vi "SendActionNum.vi"(5 "Host port":u16, 6 "RT Actions":T1 {"Slow AO Array"."Duration, Gain, NewVal" format="%#_3g"}, 7 "Host IP":string, 8 "error in (no error)":errorcluster, 9 "action #":string, 10 "Host process":string, 11 "Queue in":T5) -> (0 "error out":errorcluster)   [LabVIEW 2018]
uses:
  <vilib>/NI/AMC/Message Queue.ctl
  <vilib>/NI/AMC/Message.ctl
  <vilib>/NI/Tools/Keyed Array/KeyedArray.ctl
  RT Actions.ctl
  ActionCluster.ctl
  Instructions_RT.ctl
  ParameterSubCluster.ctl
  <vilib>/NI/AMC/Create Single Message.vi
  <vilib>/NI/AMC/Update Message Routing Info.vi
  <vilib>/NI/AMC/Send Message.vi
  <vilib>/NI/AMC/AMC.lvlib
  <vilib>/NI/Tools/Keyed Array/Tools_KeyedArray.lvlib
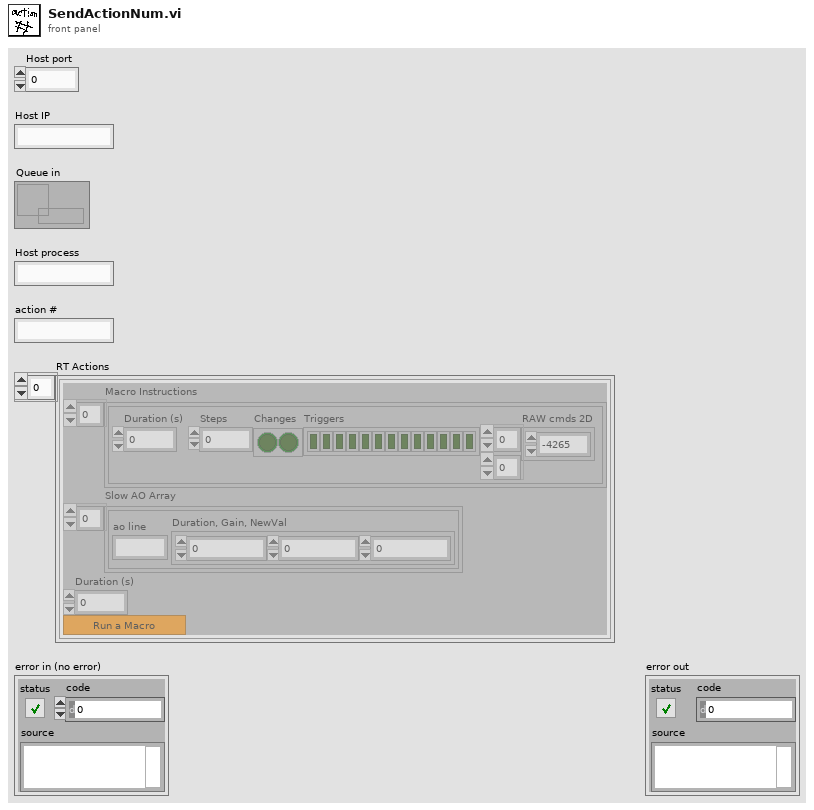
[diagram p1: front panel]
types:
  T1 = typedef "RT Actions.ctl" = T2[]
  T2 = typedef "ActionCluster.ctl" = cluster{"Macro Instructions":T3, "Slow AO Array":T4, "Duration (s)":dbl, "Toggle":bool}
  T3 = typedef "Instructions_RT.ctl" = cluster{"Duration (s)":dbl, "Steps":i32, "Changes":bool[], "Triggers":bool[], "RAW cmds 2D":i16[][]}[]
  T4 = typedef "ParameterSubCluster.ctl" = cluster{"ao line":string, "Duration, Gain, NewVal":dbl[]}[]
  T5 = typedef "AMC.lvlib/Message Queue.ctl" = refnum<queue>
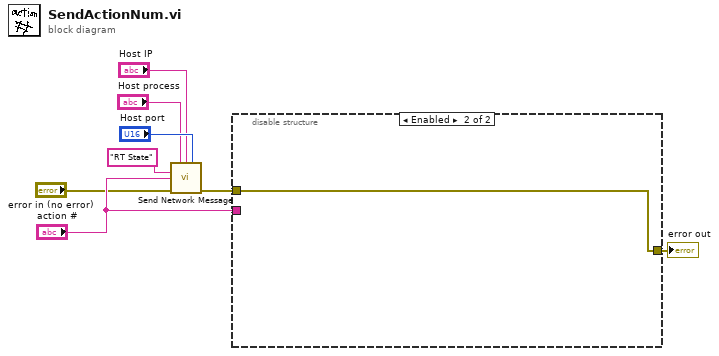
[diagram p0: block diagram]
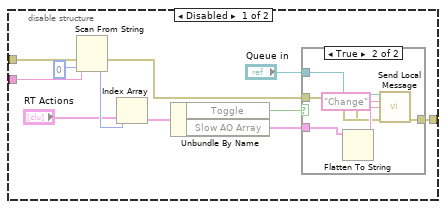
[diagram p2: hidden frame]
diagram:
  n1 = call <vilib>:"Send Network Message.vi"("receiver process"="Host process", "receiver host"="Host IP", "receiver port (0)"="Host port", "message name"="RT State", "message value"="action #", "error in"="error in (no error)") -> ("error out"=w2:errorcluster)  [unwired: 7 in, 2 out]
  n2 = disable-structure shown="Enabled" {
    disable-tunnel: "action #" -> [w19 _]
    disable-tunnel: w2 -> [w15 w27]
    disable-tunnel: [w9 w27] -> w1
    frame Disabled {
      n3 = Scan From String(input string=w19, error in=w15, default 1=u32 0 ("millisecond multiple")) -> (error out=w10:errorcluster, output 1=w18:u32)  [unwired: 2 in, 2 out]
      n4 = Index Array(array="RT Actions", index=w18) -> (element=w14:T2)
      n5 = Unbundle By Name(w14) -> ("Toggle"=w13:bool, "Slow AO Array"=w11:T4)
      n6 = case shown="True" w13 {
        tunnel: "Queue in" -> [_ w26]
        tunnel: w11 -> [_ w25]
        tunnel: w10 -> [w20 w22]
        tunnel: [w20 w21] -> _
        tunnel: [w20 w21] -> w9
        frame False {
        }
        frame True {
          n7 = Flatten To String(anything=w25) -> (data string=w24:string)  [unwired: 3 in, 2 out]
          n8 = call <vilib>:"Send Local Message.vi"("message queue in"=w26, "message name"="Change", "message value"=w24, "error in"=w22) -> ("error out"=w21:errorcluster)  [unwired: 9 in, 2 out]
        }
      }
    }
    frame Enabled {
    }
  }
  "error out" <- w1
